vi "Math SubVI - Simple (PCR) (T-CRT) (OTHER 1).vi"(1 "Input":dbl step=0.1 format="%.6f") -> (0 "Output":dbl format="%.6f")   [LabVIEW 2026]
doc: "This VI encapsulates an extremely simple mathematical operation."
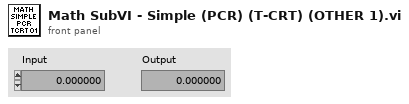
[diagram p1: front panel]
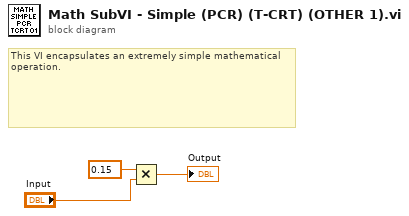
[diagram p0: block diagram]
diagram:
  # "This VI encapsulates an extremely simple mathematical operation."
  n1 = Multiply(x=0.15, y="Input") -> (x*y=→"Output":dbl)
